vi "Node Controller Stop.vi"(8 "error in (no error)":errorcluster, 11 "Simple Numeric Map Node Controller in":refnum<class "Simple Numeric Map Node Controller.lvclass">) -> (0 "error out":errorcluster, 3 "Simple Numeric Map Node Controller out":refnum<class "Simple Numeric Map Node Controller.lvclass">)   [LabVIEW 2024, in "Simple Numeric Map Node Controller.lvclass"]
uses:
  Simple Numeric Map Node Controller.lvclass
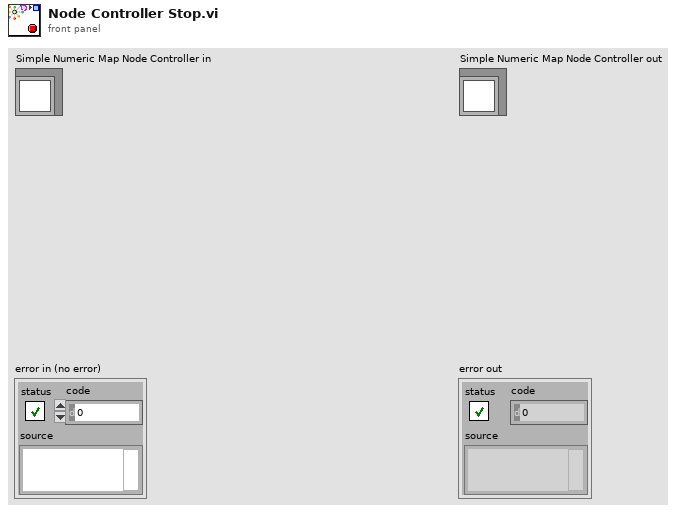
[diagram p1: front panel]
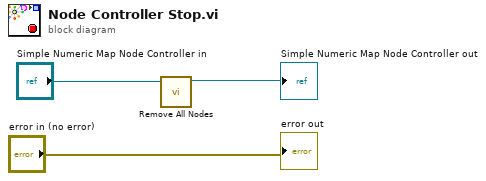
[diagram p0: block diagram]
diagram:
  n1 = call-dynamic "Remove All Nodes.vi"("Simple Numeric Map Node Controller in"="Simple Numeric Map Node Controller in") -> ("Simple Numeric Map Node Controller out"=→"Simple Numeric Map Node Controller out":refnum<class "Simple Numeric Map Node Controller.lvclass">)  [unwired: 9 in, 1 out]
  "error out" <- "error in (no error)"
